vi "Create Listener.vi"(8 "error in (no error)":errorcluster, 10 "Connection Configuration":refnum<class "Connection.lvclass">) -> (0 "error out":errorcluster, 3 "Listener":refnum<class "Connection.lvclass">)   [LabVIEW 2013, in "MQTT_Connection.lvlib" / "Connection.lvclass"]
uses:
  Connection.lvclass
  Connection.lvclass/Connection.ctl
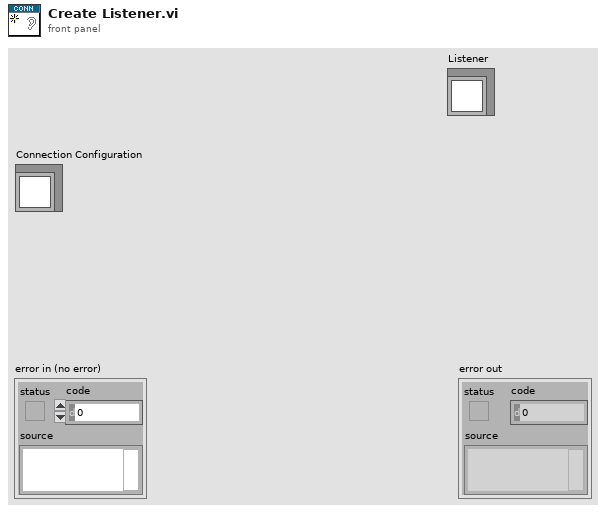
[diagram p1: front panel]
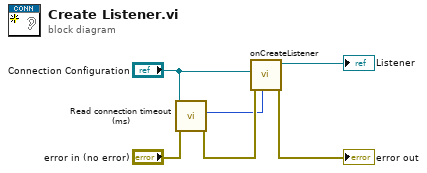
[diagram p0: block diagram]
diagram:
  n1 = call "Read connection timeout (ms).vi"("error in (no error)"="error in (no error)", "Connection in"="Connection Configuration") -> ("error out"=w3:errorcluster, "connection timeout (ms)"=w1:i32)  [unwired: 7 in, 1 out]
  n2 = call-dynamic "onCreateListener.vi"("timeout (ms)"=w1, "error in (no error)"=w3, "Configuration"="Connection Configuration") -> ("error out"=→"error out":errorcluster, "Listener"=→"Listener":refnum<class "Connection.lvclass">)  [unwired: 7 in]
